vi "SLSC Create Status.vi"() -> (3 "Outgoing configuration":T3(array[cluster])=[{"Channel Name"="LED1_Green", "SLSC Name"="Bool.LED1.NI.GreenBool", "Channel"={"Type"=enum."Input", "Units"="", "Default Value"=1.0, "Faultable"=FALSE, "Scalable"=FALSE}}, {"Channel Name"="Scratchpad8", "SLSC Name"="U32.Scratchpad8.NI.Scratchpad.AsUInt32.U8", "Channel"={"Type"=enum."Input", "Units"="", "Default Value"=12.0, "Faultable"=FALSE, "Scalable"=FALSE}}])   [LabVIEW 2015, in "SLSC-12201 DIO System Explorer.lvlib"]
uses:
  SLSC-12201 DIO System Explorer.lvlib
  <vilib>/NI Veristand/Custom Device API/Custom Device Channel.ctl
  <vilib>/NI Veristand/Custom Device API/Custom Device Channel Type.ctl
  <vilib>/NI Veristand/Custom Device API/Custom Device API.lvlib
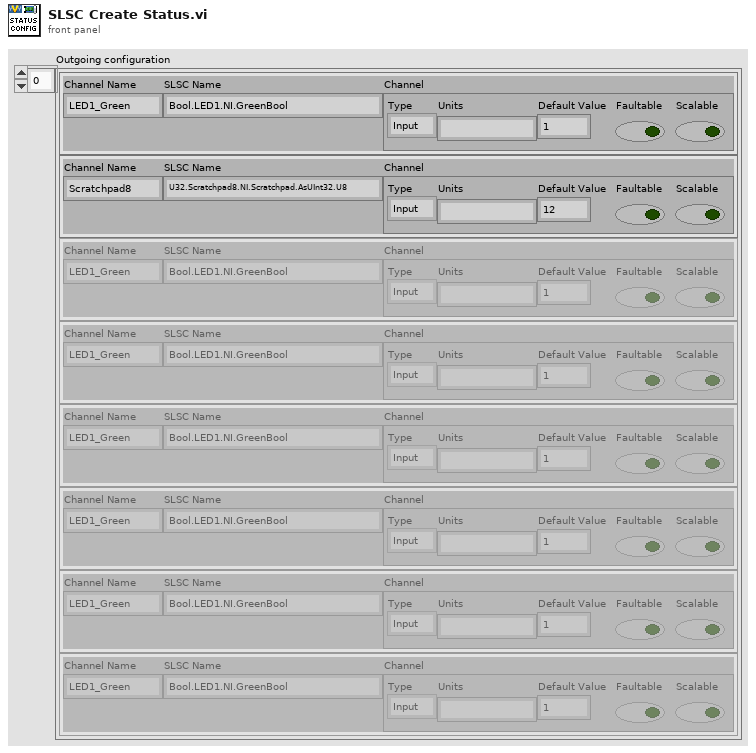
[diagram p1: front panel]
types:
  T1 = typedef "Custom Device API.lvlib/Custom Device Channel.ctl" = cluster{"Type":T2, "Units":string, "Default Value":dbl, "Faultable":bool, "Scalable":bool}
  T2 = typedef "Custom Device API.lvlib/Custom Device Channel Type.ctl" = enum16{"Input", "Output"}
  T3 = cluster{"Channel Name":string, "SLSC Name":string, "Channel":T1}[]
  T4 = cluster{"Channel Name":string, "SLSC Name":string, "Configuration":T1}[]
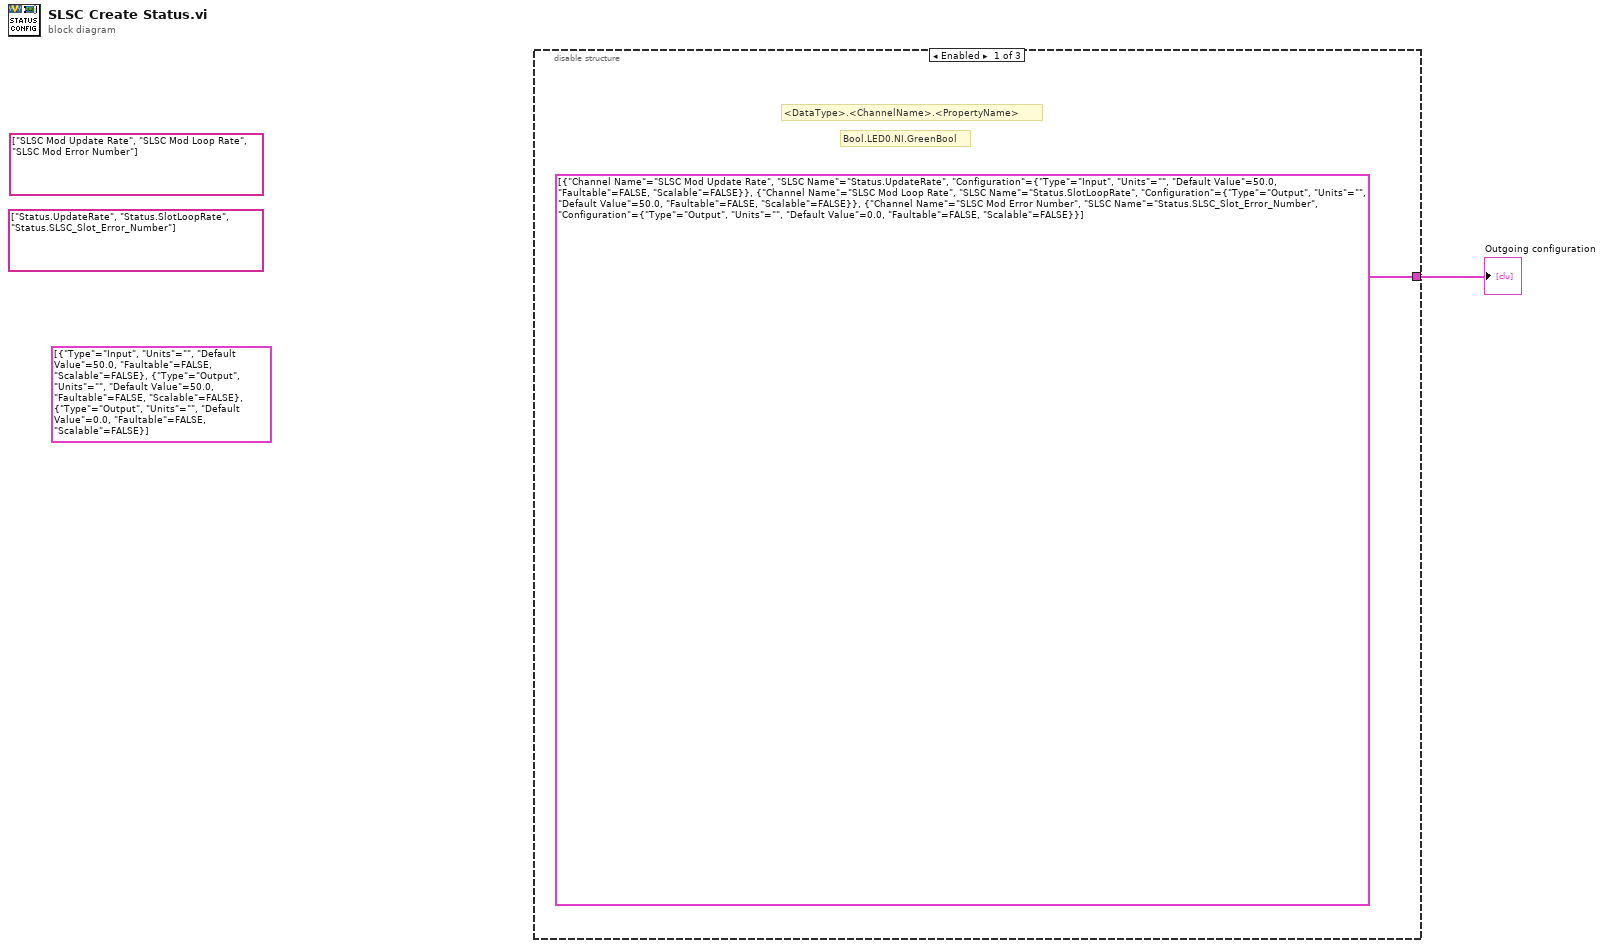
[diagram p0: block diagram]
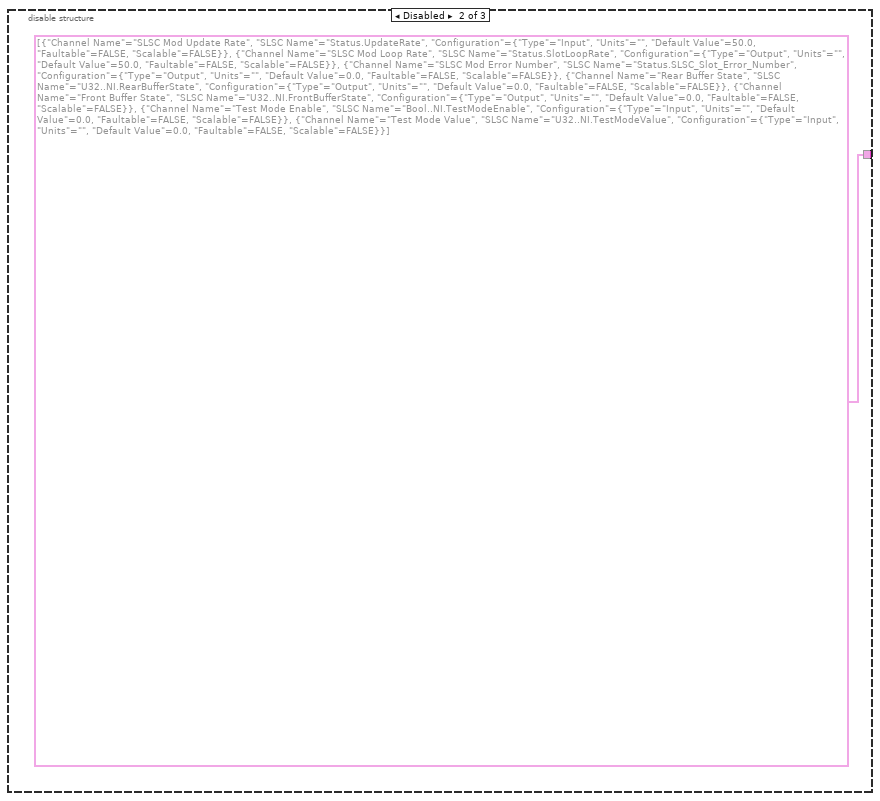
[diagram p2: hidden frame]
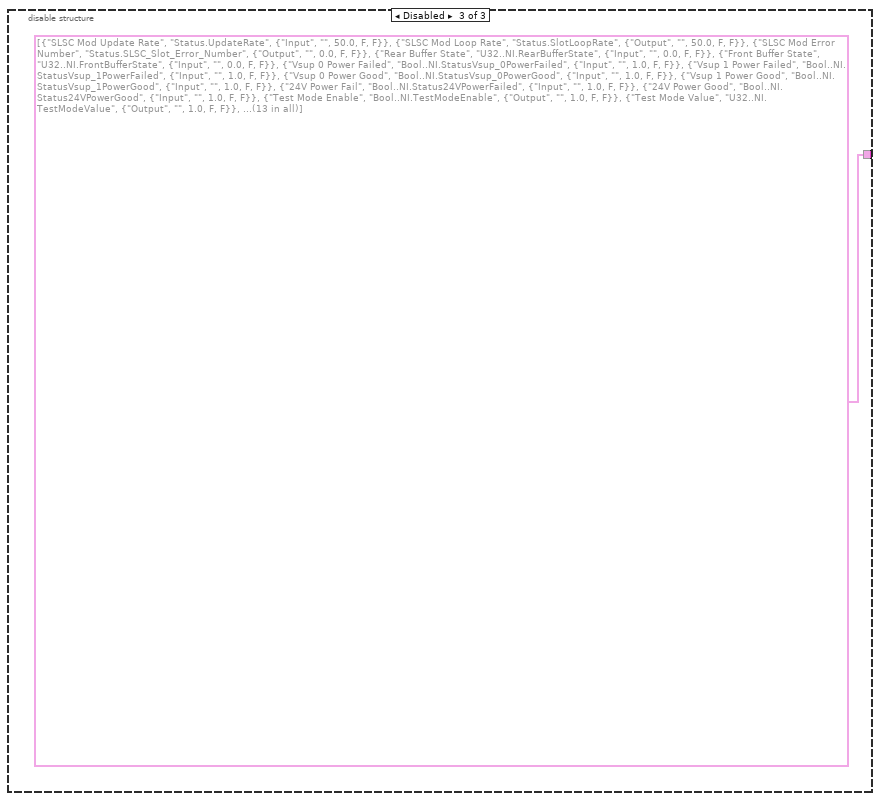
[diagram p3: hidden frame]
diagram:
  (unwired) T1[] [{"Type"=enum."Input", "Units"="", "Default Value"=50.0, "Faultable"=FALSE, "Scalable"=FALSE}, {"Type"=enum."Output", "Units"="", "Default Value"=50.0, "Faultable"=FALSE, "Scalable"=FALSE}, {"Type"=enum."Output", "Units"="", "Default Value"=0.0, "Faultable"=FALSE, "Scalable"=FALSE}]
  (unwired) string[] ["SLSC Mod Update Rate", "SLSC Mod Loop Rate", "SLSC Mod Error Number"]
  (unwired) string[] ["Status.UpdateRate", "Status.SlotLoopRate", "Status.SLSC_Slot_Error_Number"]
  n1 = disable-structure shown="Enabled" {
    disable-tunnel: [T4 [{"Channel Name"="SLSC Mod Update Rate", "SLSC Name"="Status.UpdateRate", "Configuration"={"Type"=enum."Input", "Units"="", "Default Value"=50.0, "Faultable"=FALSE, "Scalable"=FALSE}}, {"Channel Name"="SLSC Mod Loop Rate", "SLSC Name"="Status.SlotLoopRate", "Configuration"={"Type"=enum."Output", "Units"="", "Default Value"=50.0, "Faultable"=FALSE, "Scalable"=FALSE}}, {"Channel Name"="SLSC Mod Error Number", "SLSC Name"="Status.SLSC_Slot_Error_Number", "Configuration"={"Type"=enum."Output", "Units"="", "Default Value"=0.0, "Faultable"=FALSE, "Scalable"=FALSE}}] T4 [{"Channel Name"="SLSC Mod Update Rate", "SLSC Name"="Status.UpdateRate", "Configuration"={"Type"=enum."Input", "Units"="", "Default Value"=50.0, "Faultable"=FALSE, "Scalable"=FALSE}}, {"Channel Name"="SLSC Mod Loop Rate", "SLSC Name"="Status.SlotLoopRate", "Configuration"={"Type"=enum."Output", "Units"="", "Default Value"=50.0, "Faultable"=FALSE, "Scalable"=FALSE}}, {"Channel Name"="SLSC Mod Error Number", "SLSC Name"="Status.SLSC_Slot_Error_Number", "Configuration"={"Type"=enum."Output", "Units"="", "Default Value"=0.0, "Faultable"=FALSE, "Scalable"=FALSE}}, {"Channel Name"="Rear Buffer State", "SLSC Name"="U32..NI.RearBufferState", "Configuration"={"Type"=enum."Output", "Units"="", "Default Value"=0.0, "Faultable"=FALSE, "Scalable"=FALSE}}, {"Channel Name"="Front Buffer State", "SLSC Name"="U32..NI.FrontBufferState", "Configuration"={"Type"=enum."Output", "Units"="", "Default Value"=0.0, "Faultable"=FALSE, "Scalable"=FALSE}}, {"Channel Name"="Test Mode Enable", "SLSC Name"="Bool..NI.TestModeEnable", "Configuration"={"Type"=enum."Input", "Units"="", "Default Value"=0.0, "Faultable"=FALSE, "Scalable"=FALSE}}, {"Channel Name"="Test Mode Value", "SLSC Name"="U32..NI.TestModeValue", "Configuration"={"Type"=enum."Input", "Units"="", "Default Value"=0.0, "Faultable"=FALSE, "Scalable"=FALSE}}] T4 [{"Channel Name"="SLSC Mod Update Rate", "SLSC Name"="Status.UpdateRate", "Configuration"={"Type"=enum."Input", "Units"="", "Default Value"=50.0, "Faultable"=FALSE, "Scalable"=FALSE}}, {"Channel Name"="SLSC Mod Loop Rate", "SLSC Name"="Status.SlotLoopRate", "Configuration"={"Type"=enum."Output", "Units"="", "Default Value"=50.0, "Faultable"=FALSE, "Scalable"=FALSE}}, {"Channel Name"="SLSC Mod Error Number", "SLSC Name"="Status.SLSC_Slot_Error_Number", "Configuration"={"Type"=enum."Output", "Units"="", "Default Value"=0.0, "Faultable"=FALSE, "Scalable"=FALSE}}, {"Channel Name"="Rear Buffer State", "SLSC Name"="U32..NI.RearBufferState", "Configuration"={"Type"=enum."Input", "Units"="", "Default Value"=0.0, "Faultable"=FALSE, "Scalable"=FALSE}}, {"Channel Name"="Front Buffer State", "SLSC Name"="U32..NI.FrontBufferState", "Configuration"={"Type"=enum."Input", "Units"="", "Default Value"=0.0, "Faultable"=FALSE, "Scalable"=FALSE}}, {"Channel Name"="Vsup 0 Power Failed", "SLSC Name"="Bool..NI.StatusVsup_0PowerFailed", "Configuration"={"Type"=enum."Input", "Units"="", "Default Value"=1.0, "Faultable"=FALSE, "Scalable"=FALSE}}, {"Channel Name"="Vsup 1 Power Failed", "SLSC Name"="Bool..NI.StatusVsup_1PowerFailed", "Configuration"={"Type"=enum."Input", "Units"="", "Default Value"=1.0, "Faultable"=FALSE, "Scalable"=FALSE}}, {"Channel Name"="Vsup 0 Power Good", "SLSC Name"="Bool..NI.StatusVsup_0PowerGood", "Configuration"={"Type"=enum."Input", "Units"="", "Default Value"=1.0, "Faultable"=FALSE, "Scalable"=FALSE}}, {"Channel Name"="Vsup 1 Power Good", "SLSC Name"="Bool..NI.StatusVsup_1PowerGood", "Configuration"={"Type"=enum."Input", "Units"="", "Default Value"=1.0, "Faultable"=FALSE, "Scalable"=FALSE}}, {"Channel Name"="24V Power Fail", "SLSC Name"="Bool..NI.Status24VPowerFailed", "Configuration"={"Type"=enum."Input", "Units"="", "Default Value"=1.0, "Faultable"=FALSE, "Scalable"=FALSE}}, {"Channel Name"="24V Power Good", "SLSC Name"="Bool..NI.Status24VPowerGood", "Configuration"={"Type"=enum."Input", "Units"="", "Default Value"=1.0, "Faultable"=FALSE, "Scalable"=FALSE}}, {"Channel Name"="Test Mode Enable", "SLSC Name"="Bool..NI.TestModeEnable", "Configuration"={"Type"=enum."Output", "Units"="", "Default Value"=1.0, "Faultable"=FALSE, "Scalable"=FALSE}}, {"Channel Name"="Test Mode Value", "SLSC Name"="U32..NI.TestModeValue", "Configuration"={"Type"=enum."Output", "Units"="", "Default Value"=1.0, "Faultable"=FALSE, "Scalable"=FALSE}}]] -> w1
    frame Enabled {
      # "Bool.LED0.NI.GreenBool"
      # "<DataType>.<ChannelName>.<PropertyName>"
    }
    frame Disabled {
    }
    frame Disabled {
    }
  }
  "Outgoing configuration" <- w1
